vi "Memory.Pointer.Internal.Dispose.vi"(8 "error in (no error)":errorcluster, 11 "pointer":refnum<class "Memory.Pointer.Internal.lvclass">) -> (0 "error out":errorcluster)   [LabVIEW 2016, in "Memory.lvlib" / "Memory.Pointer.Internal.lvclass"]
doc: "Disposes of the provided <b>pointer</b> and deallocates the associated memory."
uses:
  Memory.Pointer.Internal.lvclass
  C:/Git/Sourcetree/DSF/Source/Submodules/Memory/Source/Classes/Pointer/Memory.Pointer.lvclass
  Pointer/Memory.Pointer.lvclass/Memory.Pointer.ctl
  Pointer/Memory.Pointer.Errors.Zone.vi
  Pointer/Memory.Pointer.Errors.Create Error.vi
  Pointer/Memory.Pointer.Errors.Null Pointer.vi
  Submodules/SEH/Source/VIs/Static Error Handling.Error Cluster Constant.vi
  Submodules/SEH/Source/VIs/Static Error Handling.Error Cluster Constant (256B).vi
  Submodules/SEH/Source/VIs/Static Error Handling.Parameters.Status.Set.vi
  Submodules/SEH/Source/VIs/Static Error Handling.Parameters.Code.Set.vi
  Submodules/SEH/Source/VIs/Static Error Handling.Parameters.VI Source.Set.vi
  Constants/Memory.Constants.vi
  Constants/Memory.Constants.Library Name.vi
  Pointer/Memory.Pointer.Errors.Get Info.vi
  Submodules/SEH/Source/VIs/Static Error Handling.Source Buffer.Write.String.vi
  Pointer/Memory.Pointer.lvclass
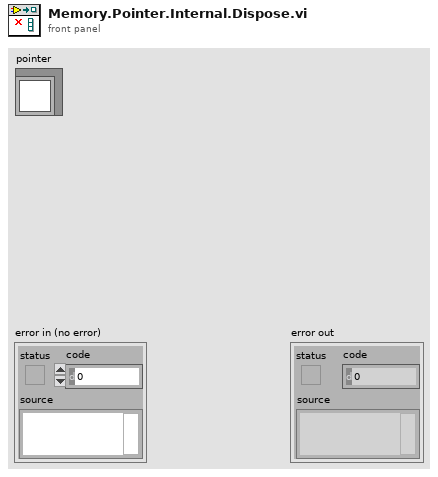
[diagram p1: front panel]
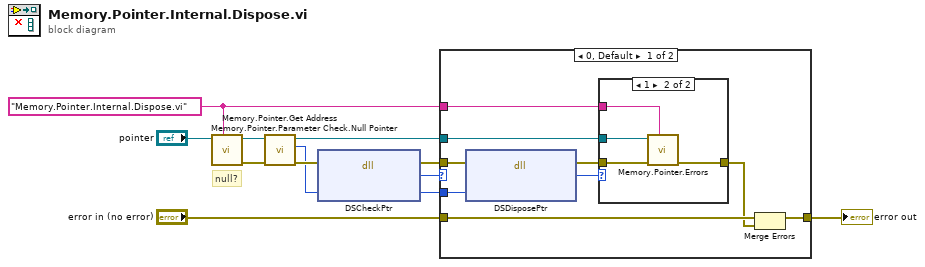
[diagram p0: block diagram]
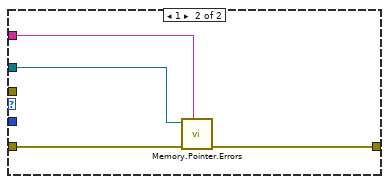
[diagram p3: hidden frame]
diagram:
  w3 = "Memory.Pointer.Internal.Dispose.vi" ("source vi name")
  # "null?"
  n1 = call "Memory.Pointer.Parameter Check.Null Pointer.vi"("source vi name"=w3, "Pointer in"="pointer") -> ("error out"=w2:errorcluster, "Pointer out"=w5:refnum<class "Memory.Pointer.Internal.lvclass">)  [unwired: 8 in]
  n2 = call "Memory.Pointer.Get Address.vi"("Pointer in"=w5) -> ("address"=w1:u64, "Pointer out"=w9:refnum<class "Memory.Pointer.Internal.lvclass">)  [unwired: 9 in]
  n3 = dll-call lib="LabVIEW" fn="DSCheckPtr"(error in=w2, "pointer"=w1) -> (error out=w10:errorcluster, "return"=w8:i32, "pointer"=w7:u64)  [unwired: 2 in, 1 out]
  n4 = case shown="0, Default" w8 {
    tunnel: [w20 w28] -> w11
    tunnel: "error in (no error)" -> [w19 w29]
    tunnel: w3 -> [w18 w27]
    tunnel: w9 -> [w14 w26]
    tunnel: w10 -> [w13 _]
    tunnel: w7 -> [w12 _]
    frame 0, Default {
      n5 = dll-call lib="LabVIEW" fn="DSDisposePtr"(error in=w13, "pointer"=w12) -> (error out=w17:errorcluster, "return"=w16:i32)  [unwired: 3 in, 1 out]
      n6 = case shown="1" w16 {
        tunnel: w17 -> [w21 w25]
        tunnel: [w21 w24] -> w15
        tunnel: w14 -> [_ w23]
        tunnel: w18 -> [_ w22]
        frame 0, Default {
        }
        frame 1 {
          n7 = call-poly "Memory.Pointer.Errors.vi"("source vi name"=w22, "error in (no error)"=w25, "pointer in"=w23) -> ("error out"=w24:errorcluster)  [unwired: 7 in, 1 out]
        }
      }
      n8 = Merge Errors(w19, w15) -> (w20:errorcluster)
    }
    frame 1 {
      n9 = call-poly "Memory.Pointer.Errors.vi"("source vi name"=w27, "error in (no error)"=w29, "pointer in"=w26) -> ("error out"=w28:errorcluster)  [unwired: 7 in, 1 out]
    }
  }
  "error out" <- w11
